vi "纳清浊度电极校准.vi"() -> ()   [LabVIEW 2016, in "斯坦道多参数.lvlib"]
uses:
  <vilib>/Utility/miscctls.llb/LVPointTypeDef.ctl
  <vilib>/Utility/miscctls.llb/LVPositionTypeDef.ctl
  <vilib>/Analysis/NI_AALBase.lvlib
panel:
  out "校准量程":u16(ring) items=["0-100", "0-500", "0-2000", "0-4000"]
  out "量程":u16(ring) items=["0-100", "0-500", "0-2000", "0-4000"]
  out "探头类别":string
  out "报警信息":string
  out "通讯状态":string
  out "温度校准参数":sgl
  out "第三点校准值":dbl
  out "标液3":sgl
  out "第二点校准值":dbl
  out "第一点校准值":dbl
  in  "校准停止":bool
  in  "校准启动":bool
  in  "校准模式":enum16{"两点校准", "单点校准", "三点校准"}(ring)=enum."单点校准"
  out "最小值":sgl format="%#.2f"
  out "最大值":sgl format="%#.2f"
  out "波形图表":u16(graph) caption="历史曲线"
  out "mean":dbl caption="均值" format="%#.2f"
  out "standard deviation":dbl caption="标准差" format="%#.2f"
  out "变异系数":dbl format="%#.6f"
  out "测量值":sgl
  out "提示":string
  out "标液2":sgl
  out "标液1":sgl
  out "原始光强数值":u16 caption="信号值"
  out "温度":dbl
  # "浊度电极设定"
  # "℃"
  # "NTU"
  # "NTU"
  # "NTU"
  # "℃"
  # "请选择校准模式:"
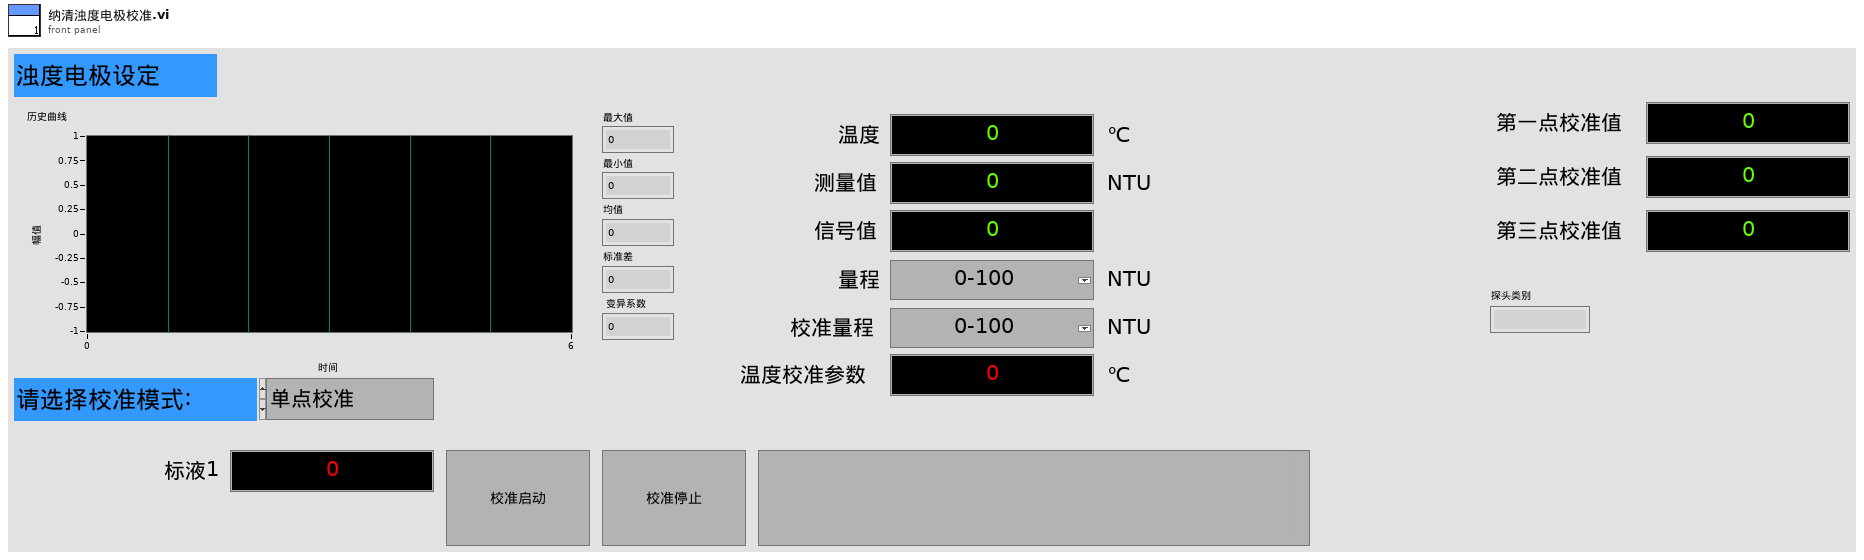
[diagram p1: front panel]
types:
  T1 = typedef "LVPointTypeDef.ctl" = cluster{"Horizontal":i16, "Vertical":i16}
  T2 = typedef "斯坦道多参数.lvlib/校准步骤.ctl" = enum16{"待机", "放置第一点标液", "第一点校准启动", "第一点校准写入", "第一点校准失败", "放置第二点标液", "第二点校准启动", "第二点校准写入", "第二点校准失败", "放置第三点标液", "第三点校准启动", "第三点校准写入", "第三点校准失败", "校准结果写入", "校准结束"}
  T3 = cluster{"报警码":u16, "浊度数值 NTU":sgl, "温度数据":sgl, "原始光强数值":u16, "量程":u16, "平均次数":u16, "清扫模式":u16, "清扫次数":u16, "清扫间隔分钟":u16, "0X000B_NC":string, "产品名称":string, "序列号":string, "硬件版本":string, "软件版本":string, "通讯地址":u16, "波特率":u16, "设备类型":u16, "0X0026_NC":string, "校准量程":u16, "第一点原始光强":u16, "第一点校准数据":sgl, "第二点原始光强":u16, "第二点校准数据":sgl, "第三点原始光强":u16, "第三点校准数据":sgl, "探头校准命令":u16, "温度校准参数":sgl, "温度校准命令":u16}
  T4 = typedef "LVPositionTypeDef.ctl" = cluster{"Left":i32, "Top":i32}
  T5 = cluster{"报警码":u16, "叶绿素a":sgl, "温度数据":sgl, "原始光强数值":u16, "0X0006_NC":u16, "平均次数":u16, "清扫模式":u16, "清扫次数":u16, "清扫间隔分钟":u16, "0X000B_NC":string, "产品名称":string, "序列号":string, "硬件版本":string, "软件版本":string, "通讯地址":u16, "波特率":u16, "设备类型":u16, "0X0026_NC":string, "0X0030_NC":u16, "第一点原始光强":u16, "第一点校准数据":sgl, "第二点原始光强":u16, "第二点校准数据":sgl, "第三点原始光强":u16, "第三点校准数据":sgl, "探头校准命令":u16, "温度校准参数":sgl, "温度校准命令":u16}
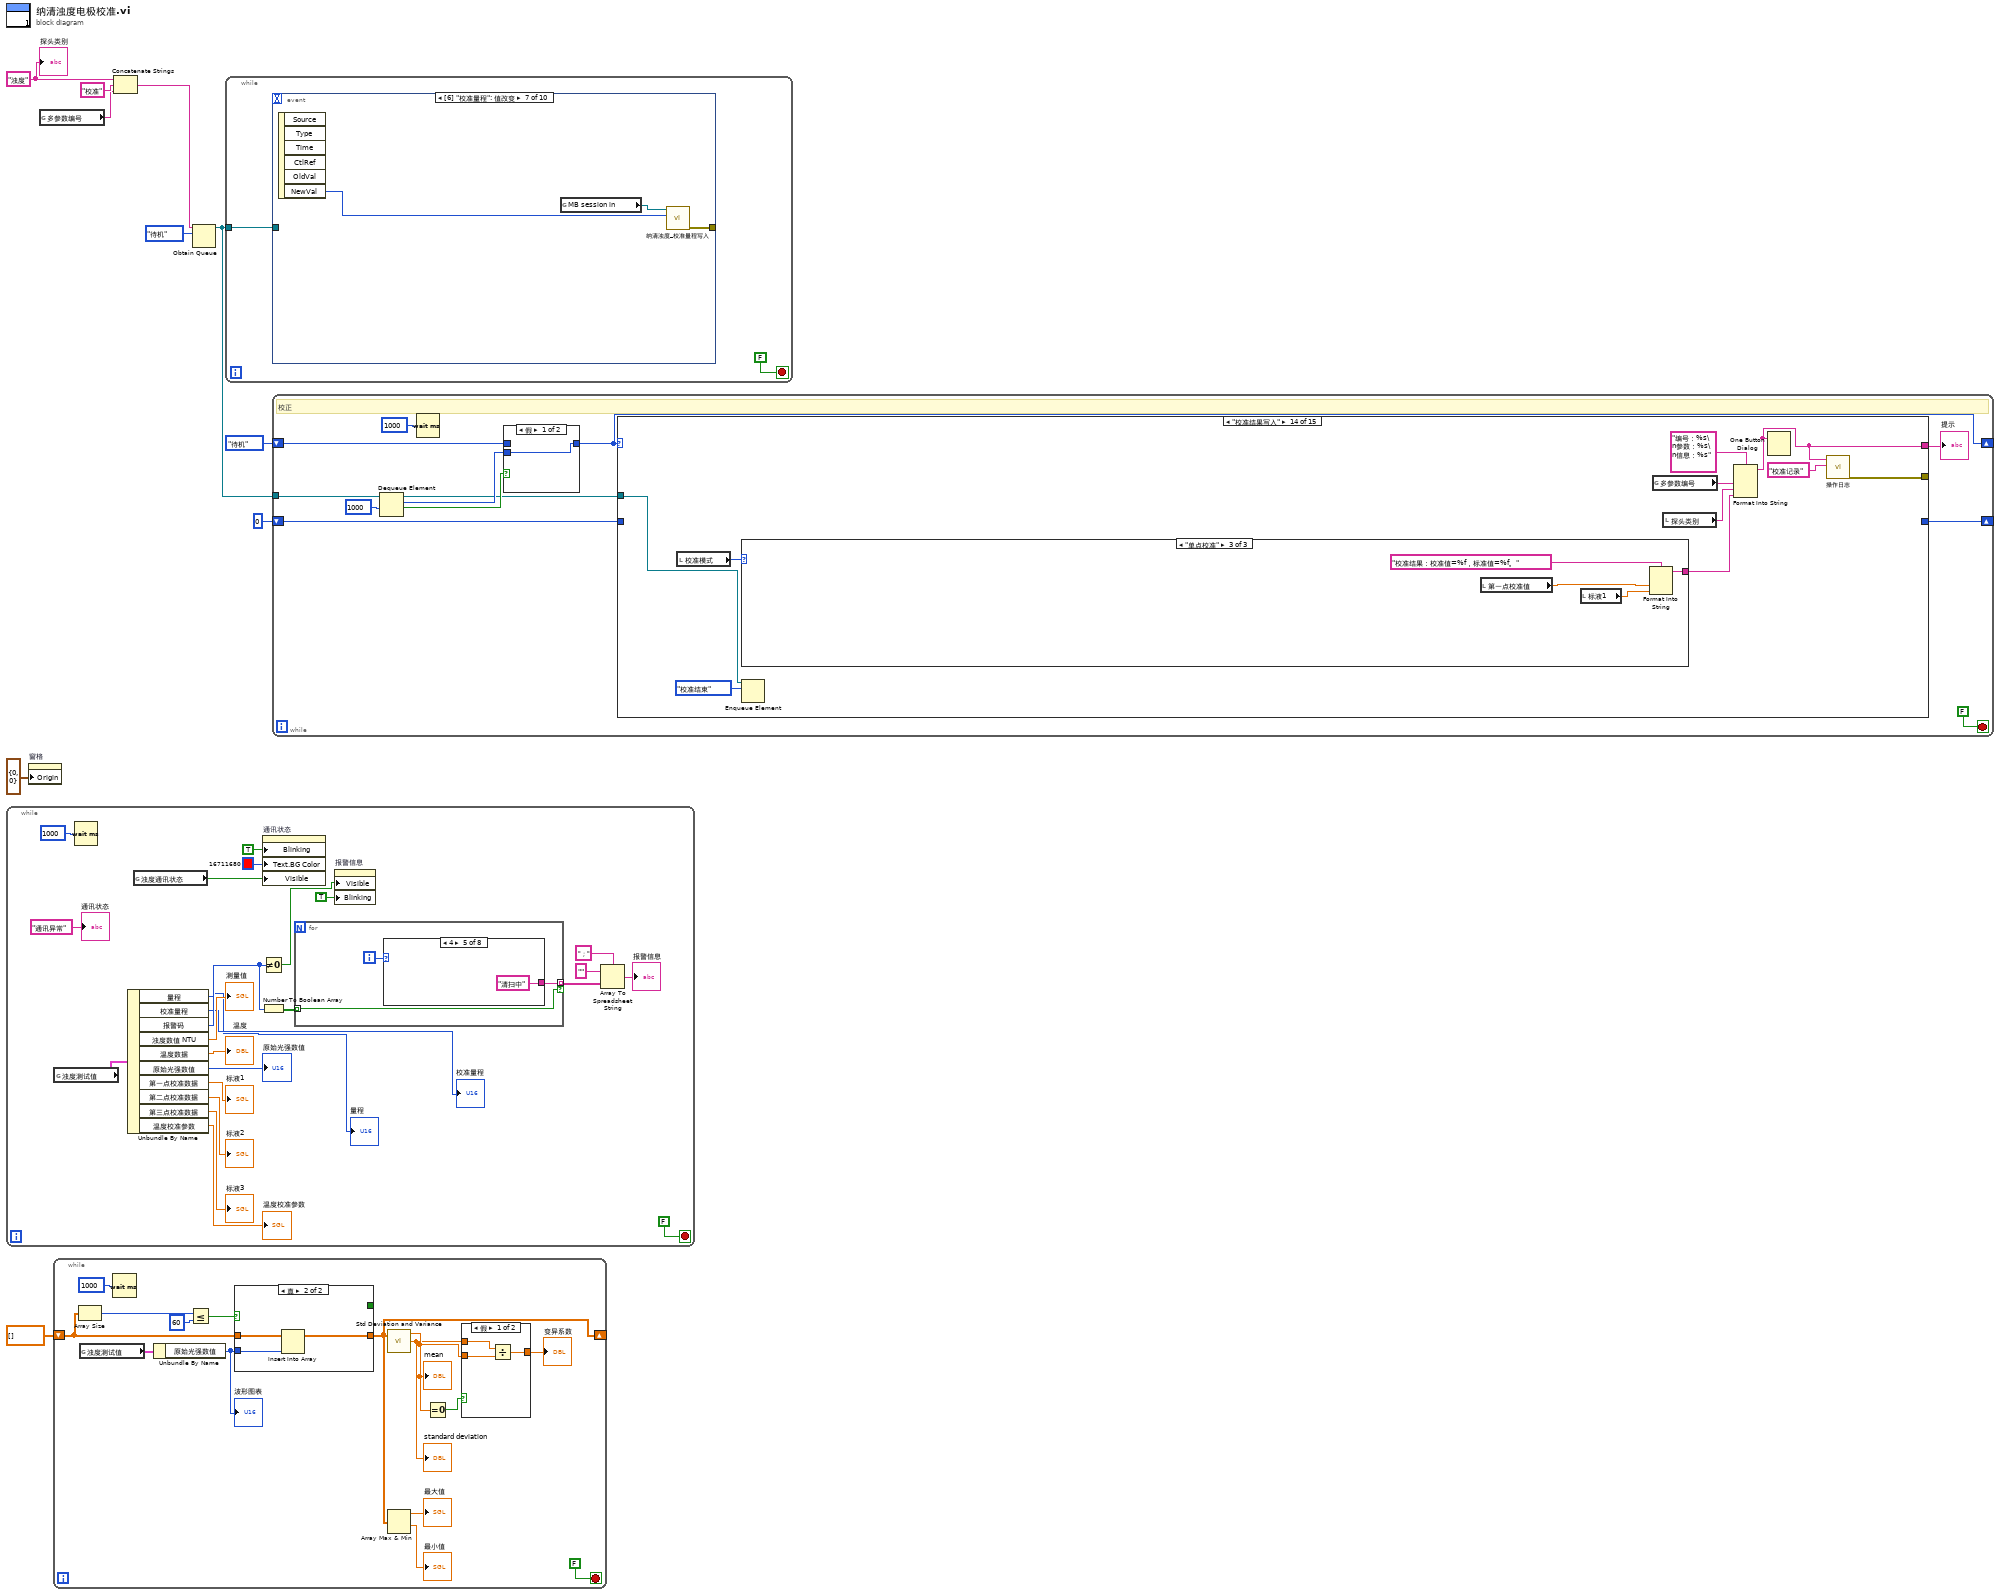
[diagram p0: block diagram]
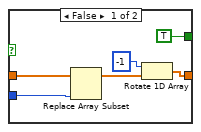
[diagram p3: hidden frame]
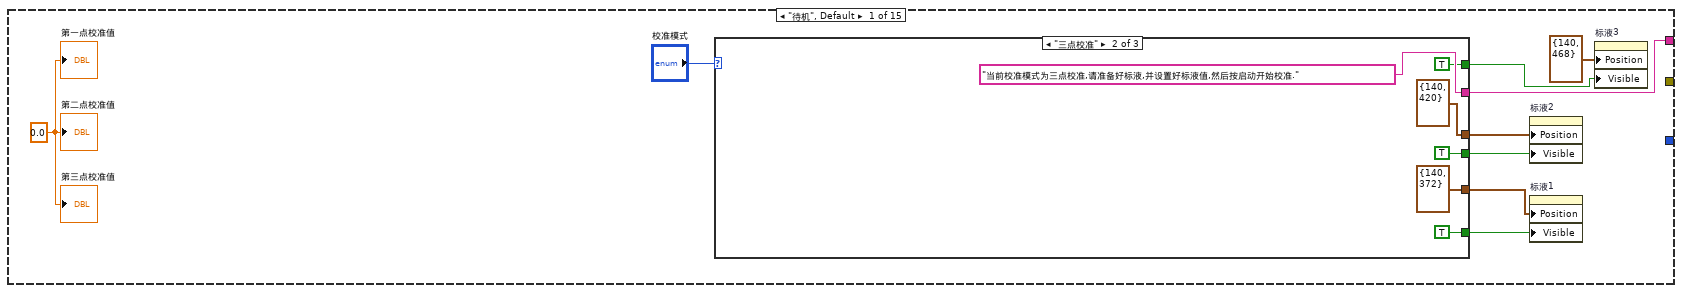
[diagram p5: hidden frame]
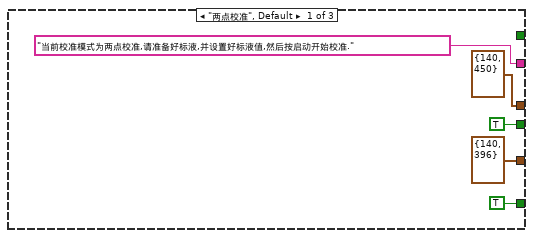
[diagram p6: hidden frame]
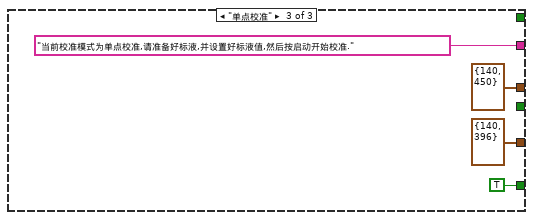
[diagram p7: hidden frame]
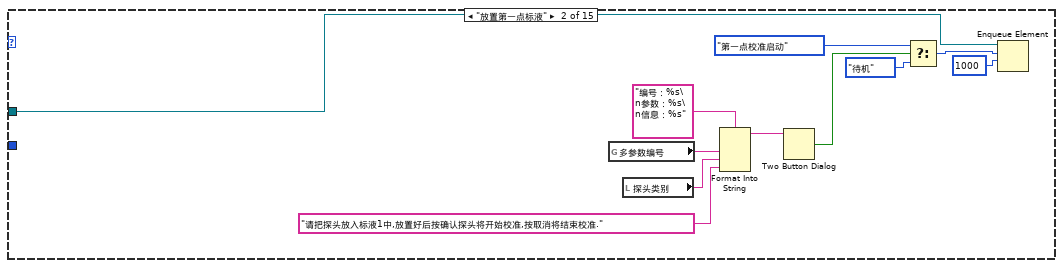
[diagram p8: hidden frame]
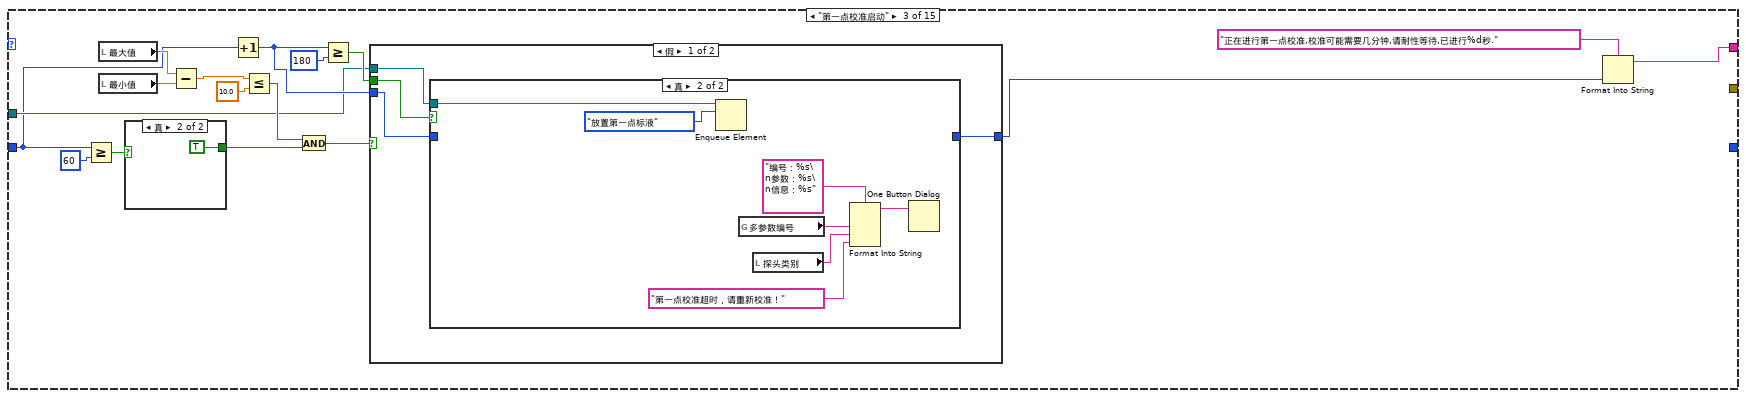
[diagram p9: hidden frame]
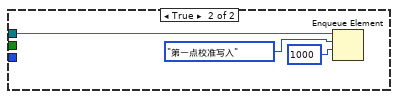
[diagram p11: hidden frame]
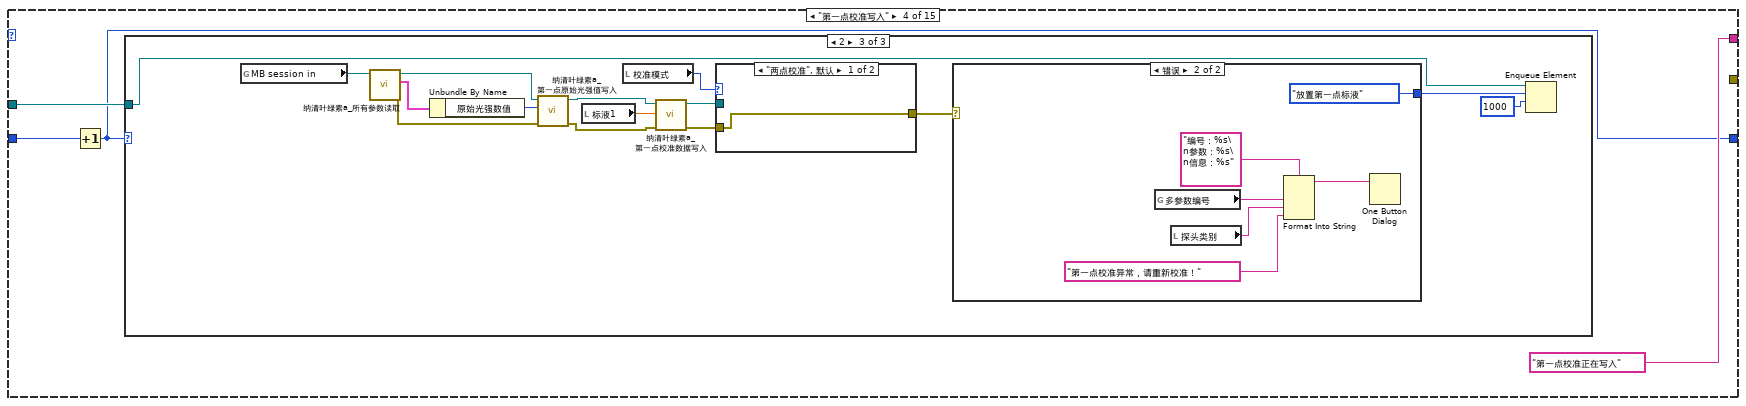
[diagram p13: hidden frame]
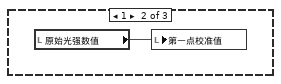
[diagram p15: hidden frame]
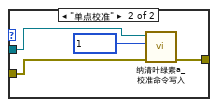
[diagram p16: hidden frame]
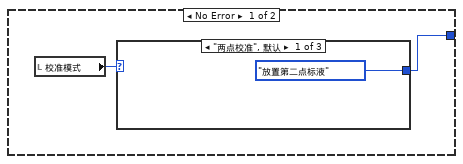
[diagram p17: hidden frame]
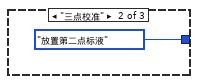
[diagram p18: hidden frame]
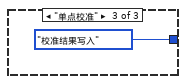
[diagram p19: hidden frame]
diagram:
  w1 = "浊度" ("名称（未命名）")
  n1 = while {
    stop <- FALSE stop-if-true
    n2 = global read "纳清过程全局变量.vi" "浊度测试值"() -> (w32:T3)
    n3 = Wait (ms)(milliseconds to wait=u32 1000 ("等待时间（毫秒）")) -> ()  [unwired: 1 out]
    n4 = Unbundle By Name(w32) -> ("量程"=→"量程":u16, "校准量程"=→"校准量程":u16, "报警码"=w13:u16, "浊度数值 NTU"=→"测量值":sgl, "温度数据"=→"温度":sgl, "原始光强数值"=→"原始光强数值":u16, "第一点校准数据"=→"标液1":sgl, "第二点校准数据"=→"标液2":sgl, "第三点校准数据"=→"标液3":sgl, "温度校准参数"=→"温度校准参数":sgl)
    n5 = global read "多参数全局变量.vi" "浊度通讯状态"() -> (w21:bool)
    n6 = Not Equal To 0?(x=w13) -> (x != 0?=w15:bool)
    n7 = Number To Boolean Array(number=w13) -> (Boolean array=w20:bool[])
    n8 = property on="通讯状态" class="Str"("Blinking"=TRUE ("闪烁"), "Text.BG Color"=u32 16711680, "Visible"=w21) -> ()  [unwired: 2 in, 2 out]
    n9 = for {
      tunnel: w20 -> [w35] mode=indexing
      tunnel: [w36] -> w19 mode=indexing if=w35
      i -> [w37]
      n10 = case shown="4" w37 {
        tunnel: [_ "浊度超量程" "温度超量程" "光强信号超范围" "清扫中" "温度传感器故障" "电极故障" "内部电压基准故障"] -> w36
        frame Default {
        }
        frame 0 {
        }
        frame 2 {
        }
        frame 3 {
        }
        frame 4 {
        }
        frame 8 {
        }
        frame 9 {
        }
        frame 10 {
        }
      }
    }
    n11 = property on="报警信息" class="Str"("Visible"=w15, "Blinking"=TRUE ("闪烁")) -> ()  [unwired: 2 in, 2 out]
    n12 = Array To Spreadsheet String(delimiter (Tab)="；" ("分隔符(Tab)"), array=w19, 3:"" ("格式字符串")) -> (spreadsheet string=→"报警信息":string)
    "通讯状态" <- "通讯异常" ("当前串口")
  }
  n13 = property on="窗格" class="Pane"("Origin"=T1 {"Horizontal"=0, "Vertical"=0} ("原点")) -> ()  [unwired: 2 in, 2 out]
  n14 = global read "多参数全局变量.vi" "多参数编号"() -> (w2:string)
  n15 = while {
    shift-right: [w49] -> _
    shift-left: sgl[] [] -> [w55]
    stop <- FALSE stop-if-true
    n16 = Array Size(array=w55) -> (size(s)=w57:i32)
    n17 = global read "纳清过程全局变量.vi" "浊度测试值"() -> (w45:T3)
    n18 = Wait (ms)(milliseconds to wait=u32 1000 ("等待时间（毫秒）")) -> ()  [unwired: 1 out]
    n19 = Unbundle By Name(w45) -> ("原始光强数值"=w46:u16)
    "波形图表" <- w46
    n20 = Less Or Equal?(x=w57, y=60) -> (x <= y?=w56:bool)
    n21 = case shown="真" w56 {
      tunnel: w55 -> [w68 w71]
      tunnel: w46 -> [w66 w70]
      tunnel: [w64 w69] -> w49
      tunnel: [TRUE _] -> _
      frame False {
        n22 = Replace Array Subset(array=w68, new element=w66) -> (w67:sgl[])  [unwired: 1 in]
        n23 = Rotate 1D Array(1:w67, 2:-1 ("n")) -> (0:w64:sgl[])
      }
      frame True {
        n24 = Insert Into Array(array=w71, new element=w70) -> (w69:sgl[])  [unwired: 1 in]
      }
    }
    n25 = call <vilib>:"Std Deviation and Variance.vi"("X"=w49) -> ("mean"=w53:dbl, "standard deviation"=w52:dbl)  [unwired: 1 in, 1 out]
    "mean" <- w53
    "standard deviation" <- w52
    n26 = Array Max & Min(array=w49) -> (max value=→"最大值":sgl, min value=→"最小值":sgl)  [unwired: 2 out]
    n27 = Equal To 0?(x=w53) -> (x = 0?=w54:bool)
    n28 = case shown="假" w54 {
      tunnel: w52 -> [w62 _]
      tunnel: [w61 _] -> w51
      tunnel: w53 -> [w60 _]
      frame False {
        n29 = Divide(x=w62, y=w60) -> (x/y=w61:dbl)
      }
      frame True {
      }
    }
    "变异系数" <- w51
  }
  n30 = Concatenate Strings(w1, "校准" ("名称（未命名）"), w2) -> (w3:string)
  n31 = Obtain Queue(name (unnamed)=w3, element data type=校准步骤."待机" ("枚举")) -> (queue out=w5:refnum<queue>)  [unwired: 3 in, 2 out]
  n32 = while {
    tunnel: w5 -> [w72]
    stop <- FALSE stop-if-true
    n33 = event shown="[6] \"校准量程\": 值改变" {
      selector: _ -> [_ _ _ _ _ _ _ _ _ _]
      dyn-events: _ -> [_ _ _ _ _ _ _ _ _ _]
      timeout: _ -> [_ _ _ _ _ _ _ _ _ _]
      tunnel: [_ _ w79 w83 w86 w89 w92 w93 _ _] -> _
      tunnel: w72 -> [_ _ _ _ _ _ _ _ w100 w102]
      event Timeout {
        n34 = event-data() -> ()  [unwired: 1 in, 3 out]
      }
      event "标液1", "标液2", "标液3", "温度校准参数": Mouse Down {
        n35 = event-data() -> ("CtlRef"=w74:refnum<vi>)  [unwired: 1 in, 7 out]
        n36 = property class="DigNum (严格)"(reference=w74) -> (reference out=w75:refnum<vi>, "Value"=w76:sgl)  [unwired: 1 in, 1 out]
        n37 = call "数字键盘.vi"("OldNumber"=w76) -> ("NewNumber"=w77:dbl)  [unwired: 1 in]
        n38 = property class="DigNum (严格)"(reference=w75, "Val(Sgnl)"=w77) -> ()  [unwired: 1 in, 2 out]
      }
      event "标液1": Value Change {
        n39 = event-data() -> ("NewVal"=w78:sgl)  [unwired: 1 in, 5 out]
        n40 = global read "多参数全局变量.vi" "MB session in"() -> (w80:refnum<class "MB_Master.lvclass">)
        n41 = call "纳清叶绿素a_第一点校准数据写入.vi"("数值"=w78, "MB session in"=w80) -> ("error out"=w79:errorcluster)  [unwired: 8 in, 1 out]
      }
      event "标液2": Value Change {
        n42 = event-data() -> ("NewVal"=w82:sgl)  [unwired: 1 in, 5 out]
        n43 = global read "多参数全局变量.vi" "MB session in"() -> (w81:refnum<class "MB_Master.lvclass">)
        n44 = call "纳清叶绿素a_第二点校准数据写入.vi"("数值"=w82, "MB session in"=w81) -> ("error out"=w83:errorcluster)  [unwired: 8 in, 1 out]
      }
      event "标液3": Value Change {
        n45 = event-data() -> ("NewVal"=w84:sgl)  [unwired: 1 in, 5 out]
        n46 = global read "多参数全局变量.vi" "MB session in"() -> (w85:refnum<class "MB_Master.lvclass">)
        n47 = call "纳清叶绿素a_第三点校准数据写入.vi"("数值"=w84, "MB session in"=w85) -> ("error out"=w86:errorcluster)  [unwired: 8 in, 1 out]
      }
      event "量程": Value Change {
        n48 = event-data() -> ("NewVal"=w87:u16)  [unwired: 1 in, 5 out]
        n49 = global read "多参数全局变量.vi" "MB session in"() -> (w88:refnum<class "MB_Master.lvclass">)
        n50 = call "纳清浊度_量程写入.vi"("数值"=w87, "MB session in"=w88) -> ("error out"=w89:errorcluster)  [unwired: 8 in, 1 out]
      }
      event "校准量程": Value Change {
        n51 = event-data() -> ("NewVal"=w90:u16)  [unwired: 1 in, 5 out]
        n52 = global read "多参数全局变量.vi" "MB session in"() -> (w91:refnum<class "MB_Master.lvclass">)
        n53 = call "纳清浊度_校准量程写入.vi"("数值"=w90, "MB session in"=w91) -> ("error out"=w92:errorcluster)  [unwired: 8 in, 1 out]
      }
      event "温度校准参数": Value Change {
        n54 = event-data() -> ("NewVal"=w98:sgl)  [unwired: 1 in, 5 out]
        n55 = global read "多参数全局变量.vi" "MB session in"() -> (w97:refnum<class "MB_Master.lvclass">)
        n56 = call "纳清叶绿素a_温度校准参数写入.vi"("数值"=w98, "MB session in"=w97) -> ("error out"=w99:errorcluster, "MB session out"=w96:refnum<class "MB_Master.lvclass">)  [unwired: 8 in]
        n57 = call "纳清叶绿素a_温度校准命令写入.vi"("error in (no error)"=w99, "数值"=u16 1 ("starting address"), "MB session in"=w96) -> ("error out"=w94:errorcluster)  [unwired: 7 in, 1 out]
        n58 = call <vilib>:"Simple Error Handler.vi"("error in (no error)"=w94) -> ("error out"=w93:errorcluster)  [unwired: 4 in, 4 out]
      }
      event "校准启动": Value Change {
        n59 = event-data() -> ()  [unwired: 1 in, 6 out]
        n60 = Enqueue Element(queue=w100, element=校准步骤."放置第一点标液" ("元素")) -> ()  [unwired: 2 in, 3 out]
      }
      event "校准停止": Value Change {
        n61 = event-data() -> ()  [unwired: 1 in, 6 out]
        n62 = Flush Queue(queue=w102) -> (queue out=w103:refnum<queue>)  [unwired: 1 in, 2 out]
        n63 = Enqueue Element(queue=w103, element=校准步骤."待机" ("元素"), timeout in ms (-1)=1000 ("超时毫秒(-1)")) -> ()  [unwired: 1 in, 3 out]
      }
    }
  }
  n64 = while "While循环" {
    shift-right: [w107] -> _
    shift-left: 校准步骤."待机" ("枚举") -> [w109]
    shift-right: [w106] -> _
    shift-left: 0 -> [w115]
    tunnel: w5 -> [w110]
    stop <- FALSE stop-if-true
    # "校正"
    n65 = Dequeue Element(queue=w110, timeout in ms (-1)=1000 ("超时毫秒(-1)")) -> (queue out=w108:refnum<queue>, element=w111:T2, timed out?=w112:bool)  [unwired: 1 in, 1 out]
    n66 = Wait (ms)(milliseconds to wait=u32 1000 ("等待时间（毫秒）")) -> ()  [unwired: 1 out]
    n67 = case shown="假" w112 {
      tunnel: w111 -> [w118 _]
      tunnel: [w118 w119] -> w107
      tunnel: w109 -> [_ w119]
      frame False {
      }
      frame True {
      }
    }
    n68 = case shown="\"校准结果写入\"" w107 {
      tunnel: [w127 _ w155 "第一点校准正在写入" ("提示") _ _ w237 "第二点校准正在写入" ("提示") "第二点校准失败" ("提示") _ "第三点校准正在写入" ("提示") w349 "第三点校准失败" ("提示") w383 w409] -> w114
      tunnel: w115 -> [_ _ w157 w190 _ _ w238 w270 _ _ w318 w350 _ _ _]
      tunnel: [_ _ _ w188 _ _ w236 w268 _ _ w316 w348 _ _ _] -> w106
      tunnel: w108 -> [_ w150 w158 w189 _ w229 w239 w269 _ w310 w317 w351 _ w389 _]
      tunnel: [_ _ _ _ _ _ _ _ _ _ _ _ _ w387 _] -> _
      frame "待机", Default {
        w120 = 0.0 ("第一点校准值")
        n69 = case shown="\"三点校准\"" "校准模式" {
          tunnel: ["当前校准模式为两点校准,请准备好标液,并设置好标液值,然后按启动开始校准." ("提示") "当前校准模式为三点校准,请准备好标液,并设置好标液值,然后按启动开始校准." ("提示") "当前校准模式为单点校准,请准备好标液,并设置好标液值,然后按启动开始校准." ("提示")] -> w127
          tunnel: [TRUE ("可见") TRUE ("可见") _] -> w123
          tunnel: [T4 {"Left"=140, "Top"=396} ("位置") T4 {"Left"=140, "Top"=372} ("位置") T4 {"Left"=140, "Top"=396} ("位置")] -> w126
          tunnel: [T4 {"Left"=140, "Top"=450} ("位置 2") T4 {"Left"=140, "Top"=420} ("位置 2") T4 {"Left"=140, "Top"=450} ("位置 2")] -> w125
          tunnel: [_ TRUE ("可见") _] -> w122
          tunnel: [TRUE ("可见") TRUE ("可见") TRUE ("可见")] -> w121
          frame "两点校准", Default {
          }
          frame "三点校准" {
          }
          frame "单点校准" {
          }
        }
        n70 = property on="标液2" class="DigNum (严格)"("Position"=w125, "Visible"=w123) -> ()  [unwired: 2 in, 2 out]
        n71 = property on="标液1" class="DigNum (严格)"("Position"=w126, "Visible"=w121) -> ()  [unwired: 2 in, 2 out]
        n72 = property on="标液3" class="DigNum (严格)"("Position"=T4 {"Left"=140, "Top"=468} ("位置 3"), "Visible"=w122) -> ()  [unwired: 2 in, 2 out]
        "第一点校准值" <- w120
        "第二点校准值" <- w120
        "第三点校准值" <- w120
      }
      frame "放置第一点标液" {
        n73 = global read "多参数全局变量.vi" "多参数编号"() -> (w148:string)
        n74 = local read "探头类别"() -> (w144:string)
        n75 = Format Into String(format string="编号：%s\n参数：%s\n信息：%s" ("格式字符串"), w148, w144, "请把探头放入标液1中,放置好后按确认探头将开始校准,按取消将结束校准." ("消息")) -> (resulting string=w147:string)  [unwired: 2 in, 1 out]
        n76 = Two Button Dialog(message=w147) -> (T button?=w145:bool)  [unwired: 2 in]
        n77 = Select(t=校准步骤."第一点校准启动" ("元素"), s=w145, f=校准步骤."待机" ("元素")) -> (s? t:f=w151:T2)
        n78 = Enqueue Element(queue=w150, element=w151, timeout in ms (-1)=1000 ("超时毫秒(-1)")) -> ()  [unwired: 1 in, 3 out]
      }
      frame "第一点校准启动" {
        n79 = Greater Or Equal?(x=w157, y=60) -> (x >= y?=w164:bool)
        n80 = local read "最大值"() -> (w167:sgl)
        n81 = local read "最小值"() -> (w166:sgl)
        n82 = case shown="真" w164 {
          tunnel: [_ TRUE] -> w165
          frame False {
          }
          frame True {
          }
        }
        n83 = Subtract(x=w167, y=w166) -> (x-y=w168:sgl)
        n84 = Increment(x=w157) -> (x+1=w171:i32)
        n85 = Less Or Equal?(x=w168, y=10.0) -> (x <= y?=w161:bool)
        n86 = And(x=w161, y=w165) -> (x .and. y?=w169:bool)
        n87 = Greater Or Equal?(x=w171, y=180) -> (x >= y?=w170:bool)
        n88 = case shown="假" w169 {
          tunnel: w158 -> [w174 w186]
          tunnel: w170 -> [w175 _]
          tunnel: w171 -> [w173 _]
          tunnel: [w172 _] -> w156
          frame False {
            n89 = case shown="真" w175 {
              tunnel: w174 -> [_ w183]
              tunnel: w173 -> [w176 _]
              tunnel: [w176 _] -> w172
              frame False {
              }
              frame True {
                n90 = Enqueue Element(queue=w183, element=校准步骤."放置第一点标液" ("元素")) -> ()  [unwired: 2 in, 3 out]
                n91 = global read "多参数全局变量.vi" "多参数编号"() -> (w180:string)
                n92 = local read "探头类别"() -> (w177:string)
                n93 = Format Into String(format string="编号：%s\n参数：%s\n信息：%s" ("格式字符串"), w180, w177, "第一点校准超时，请重新校准！" ("error source (\" \")")) -> (resulting string=w178:string)  [unwired: 2 in, 1 out]
                n94 = One Button Dialog(message=w178) -> ()  [unwired: 1 in, 1 out]
              }
            }
          }
          frame True {
            n95 = Enqueue Element(queue=w186, element=校准步骤."第一点校准写入" ("元素"), timeout in ms (-1)=1000 ("超时毫秒(-1)")) -> ()  [unwired: 1 in, 3 out]
          }
        }
        n96 = Format Into String(format string="正在进行第一点校准,校准可能需要几分钟,请耐性等待,已进行%d秒." ("格式字符串"), w156) -> (resulting string=w155:string)  [unwired: 2 in, 1 out]
      }
      frame "第一点校准写入" {
        n97 = Increment(x=w190) -> (x+1=w188:i32)
        n98 = case shown="2" w188 {
          tunnel: w189 -> [_ _ w207]
          frame 0, Default {
          }
          frame 1 {
            n99 = local read "原始光强数值"() -> (w192:u16)
            n100 = local write "第一点校准值"(w192) -> ()
          }
          frame 2 {
            n101 = global read "多参数全局变量.vi" "MB session in"() -> (w203:refnum<class "MB_Master.lvclass">)
            n102 = call "纳清叶绿素a_所有参数读取.vi"("MB session in"=w203) -> ("error out"=w205:errorcluster, "输出值"=w202:T5, "MB session out"=w204:refnum<class "MB_Master.lvclass">)  [unwired: 8 in]
            n103 = Unbundle By Name(w202) -> ("原始光强数值"=w201:u16)
            n104 = call "纳清叶绿素a_第一点原始光强值写入.vi"("error in (no error)"=w205, "数值"=w201, "MB session in"=w204) -> ("error out"=w200:errorcluster, "MB session out"=w199:refnum<class "MB_Master.lvclass">)  [unwired: 7 in]
            n105 = local read "标液1"() -> (w196:sgl)
            n106 = local read "校准模式"() -> (w193:enum16{"两点校准", "单点校准", "三点校准"})
            n107 = call "纳清叶绿素a_第一点校准数据写入.vi"("error in (no error)"=w200, "数值"=w196, "MB session in"=w199) -> ("error out"=w198:errorcluster, "MB session out"=w197:refnum<class "MB_Master.lvclass">)  [unwired: 7 in]
            n108 = case shown="\"两点校准\", 默认" w193 {
              tunnel: w198 -> [w208 w212]
              tunnel: w197 -> [_ w211]
              tunnel: [w208 w209] -> w195
              frame "两点校准", Default {
              }
              frame "单点校准" {
                n109 = call "纳清叶绿素a_校准命令写入.vi"("error in (no error)"=w212, "数值"=u16 1 ("starting address"), "MB session in"=w211) -> ("error out"=w209:errorcluster)  [unwired: 7 in, 1 out]
              }
            }
            n110 = case shown="错误" w195 {
              tunnel: [w213 校准步骤."放置第一点标液" ("元素")] -> w194
              frame No Error {
                n111 = local read "校准模式"() -> (w214:enum16{"两点校准", "单点校准", "三点校准"})
                n112 = case shown="\"两点校准\", 默认" w214 {
                  tunnel: [校准步骤."放置第二点标液" ("元素") 校准步骤."放置第二点标液" ("元素") 校准步骤."校准结果写入" ("元素")] -> w213
                  frame "两点校准", Default {
                  }
                  frame "三点校准" {
                  }
                  frame "单点校准" {
                  }
                }
              }
              frame Error {
                n113 = global read "多参数全局变量.vi" "多参数编号"() -> (w222:string)
                n114 = local read "探头类别"() -> (w218:string)
                n115 = Format Into String(format string="编号：%s\n参数：%s\n信息：%s" ("格式字符串"), w222, w218, "第一点校准异常，请重新校准！" ("error source (\" \")")) -> (resulting string=w220:string)  [unwired: 2 in, 1 out]
                n116 = One Button Dialog(message=w220) -> ()  [unwired: 1 in, 1 out]
              }
            }
            n117 = Enqueue Element(queue=w207, element=w194, timeout in ms (-1)=1000 ("超时毫秒(-1)")) -> ()  [unwired: 1 in, 3 out]
          }
        }
      }
      frame "第一点校准失败" {
      }
      frame "放置第二点标液" {
        n118 = global read "多参数全局变量.vi" "多参数编号"() -> (w227:string)
        n119 = local read "探头类别"() -> (w224:string)
        n120 = Format Into String(format string="编号：%s\n参数：%s\n信息：%s" ("格式字符串"), w227, w224, "请把探头放入标液2中,放置好后按确认将继续校准,按取消将结束校准." ("消息")) -> (resulting string=w226:string)  [unwired: 2 in, 1 out]
        n121 = Two Button Dialog(message=w226) -> (T button?=w233:bool)  [unwired: 2 in]
        n122 = Select(t=校准步骤."第二点校准启动" ("元素"), s=w233, f=校准步骤."待机" ("元素")) -> (s? t:f=w230:T2)
        n123 = Enqueue Element(queue=w229, element=w230, timeout in ms (-1)=1000 ("超时毫秒(-1)")) -> ()  [unwired: 1 in, 3 out]
      }
      frame "第二点校准启动" {
        n124 = Greater Or Equal?(x=w238, y=60) -> (x >= y?=w244:bool)
        n125 = local read "最大值"() -> (w247:sgl)
        n126 = local read "最小值"() -> (w246:sgl)
        n127 = case shown="真" w244 {
          tunnel: [_ TRUE] -> w245
          frame False {
          }
          frame True {
          }
        }
        n128 = Subtract(x=w247, y=w246) -> (x-y=w248:sgl)
        n129 = Increment(x=w238) -> (x+1=w251:i32)
        n130 = Less Or Equal?(x=w248, y=10.0) -> (x <= y?=w241:bool)
        n131 = And(x=w241, y=w245) -> (x .and. y?=w249:bool)
        n132 = Greater Or Equal?(x=w251, y=180) -> (x >= y?=w250:bool)
        n133 = case shown="假" w249 {
          tunnel: w239 -> [w254 w266]
          tunnel: w250 -> [w255 _]
          tunnel: w251 -> [w253 _]
          tunnel: [w252 _] -> w236
          frame False {
            n134 = case shown="真" w255 {
              tunnel: w254 -> [_ w263]
              tunnel: w253 -> [w256 _]
              tunnel: [w256 _] -> w252
              frame False {
              }
              frame True {
                n135 = Enqueue Element(queue=w263, element=校准步骤."放置第二点标液" ("元素")) -> ()  [unwired: 2 in, 3 out]
                n136 = global read "多参数全局变量.vi" "多参数编号"() -> (w260:string)
                n137 = local read "探头类别"() -> (w257:string)
                n138 = Format Into String(format string="编号：%s\n参数：%s\n信息：%s" ("格式字符串"), w260, w257, "第二点校准超时，请重新校准！" ("消息")) -> (resulting string=w259:string)  [unwired: 2 in, 1 out]
                n139 = One Button Dialog(message=w259) -> ()  [unwired: 1 in, 1 out]
              }
            }
          }
          frame True {
            n140 = Enqueue Element(queue=w266, element=校准步骤."第二点校准写入" ("元素"), timeout in ms (-1)=1000 ("超时毫秒(-1)")) -> ()  [unwired: 1 in, 3 out]
          }
        }
        n141 = Format Into String(format string="正在进行第二点校准,校准可能需要几分钟,请耐性等待,已进行%d秒." ("格式字符串"), w236) -> (resulting string=w237:string)  [unwired: 2 in, 1 out]
      }
      frame "第二点校准写入" {
        n142 = Increment(x=w270) -> (x+1=w268:i32)
        n143 = case shown="2" w268 {
          tunnel: w269 -> [_ _ w287]
          frame 0, Default {
          }
          frame 1 {
            n144 = local read "原始光强数值"() -> (w272:u16)
            n145 = local write "第二点校准值"(w272) -> ()
          }
          frame 2 {
            n146 = global read "多参数全局变量.vi" "MB session in"() -> (w283:refnum<class "MB_Master.lvclass">)
            n147 = call "纳清叶绿素a_所有参数读取.vi"("MB session in"=w283) -> ("error out"=w285:errorcluster, "输出值"=w282:T5, "MB session out"=w284:refnum<class "MB_Master.lvclass">)  [unwired: 8 in]
            n148 = Unbundle By Name(w282) -> ("原始光强数值"=w281:u16)
            n149 = call "纳清叶绿素a_第二点原始光强值写入.vi"("error in (no error)"=w285, "数值"=w281, "MB session in"=w284) -> ("error out"=w280:errorcluster, "MB session out"=w279:refnum<class "MB_Master.lvclass">)  [unwired: 7 in]
            n150 = local read "标液2"() -> (w276:sgl)
            n151 = local read "校准模式"() -> (w273:enum16{"两点校准", "单点校准", "三点校准"})
            n152 = call "纳清叶绿素a_第二点校准数据写入.vi"("error in (no error)"=w280, "数值"=w276, "MB session in"=w279) -> ("error out"=w278:errorcluster, "MB session out"=w277:refnum<class "MB_Master.lvclass">)  [unwired: 7 in]
            n153 = case shown="\"单点校准\", 默认" w273 {
              tunnel: w278 -> [w291 w292]
              tunnel: w277 -> [w290 _]
              tunnel: [w288 w292] -> w275
              frame "两点校准" {
                n154 = call "纳清叶绿素a_校准命令写入.vi"("error in (no error)"=w291, "数值"=u16 2 ("starting address"), "MB session in"=w290) -> ("error out"=w288:errorcluster)  [unwired: 7 in, 1 out]
              }
              frame "单点校准", Default {
              }
            }
            n155 = case shown="错误" w275 {
              tunnel: [w293 校准步骤."放置第二点标液" ("元素")] -> w274
              frame No Error {
                n156 = local read "校准模式"() -> (w294:enum16{"两点校准", "单点校准", "三点校准"})
                n157 = case shown="\"两点校准\", 默认" w294 {
                  tunnel: [校准步骤."校准结果写入" ("元素") 校准步骤."放置第三点标液" ("元素") 校准步骤."校准结果写入" ("元素")] -> w293
                  frame "两点校准", Default {
                  }
                  frame "三点校准" {
                  }
                  frame "单点校准" {
                  }
                }
              }
              frame Error {
                n158 = global read "多参数全局变量.vi" "多参数编号"() -> (w302:string)
                n159 = local read "探头类别"() -> (w298:string)
                n160 = Format Into String(format string="编号：%s\n参数：%s\n信息：%s" ("格式字符串"), w302, w298, "第二点校准异常，请重新校准！" ("error source (\" \")")) -> (resulting string=w300:string)  [unwired: 2 in, 1 out]
                n161 = One Button Dialog(message=w300) -> ()  [unwired: 1 in, 1 out]
              }
            }
            n162 = Enqueue Element(queue=w287, element=w274, timeout in ms (-1)=1000 ("超时毫秒(-1)")) -> ()  [unwired: 1 in, 3 out]
          }
        }
      }
      frame "第二点校准失败" {
      }
      frame "放置第三点标液" {
        n163 = global read "多参数全局变量.vi" "多参数编号"() -> (w308:string)
        n164 = local read "探头类别"() -> (w305:string)
        n165 = Format Into String(format string="编号：%s\n参数：%s\n信息：%s" ("格式字符串"), w308, w305, "请把探头放入标液3中,放置好后按确认将继续校准,按取消将结束校准." ("消息")) -> (resulting string=w307:string)  [unwired: 2 in, 1 out]
        n166 = Two Button Dialog(message=w307) -> (T button?=w314:bool)  [unwired: 2 in]
        n167 = Select(t=校准步骤."第三点校准启动" ("元素"), s=w314, f=校准步骤."待机" ("元素")) -> (s? t:f=w311:T2)
        n168 = Enqueue Element(queue=w310, element=w311, timeout in ms (-1)=1000 ("超时毫秒(-1)")) -> ()  [unwired: 1 in, 3 out]
      }
      frame "第三点校准写入" {
        n169 = Increment(x=w318) -> (x+1=w316:i32)
        n170 = case shown="2" w316 {
          tunnel: w317 -> [_ _ w322]
          frame 0, Default {
          }
          frame 1 {
            n171 = local read "原始光强数值"() -> (w320:u16)
            n172 = local write "第二点校准值"(w320) -> ()
          }
          frame 2 {
            n173 = global read "多参数全局变量.vi" "MB session in"() -> (w333:refnum<class "MB_Master.lvclass">)
            n174 = call "纳清叶绿素a_所有参数读取.vi"("MB session in"=w333) -> ("error out"=w335:errorcluster, "输出值"=w332:T5, "MB session out"=w334:refnum<class "MB_Master.lvclass">)  [unwired: 8 in]
            n175 = Unbundle By Name(w332) -> ("原始光强数值"=w331:u16)
            n176 = call "纳清叶绿素a_第三点原始光强值写入.vi"("error in (no error)"=w335, "数值"=w331, "MB session in"=w334) -> ("error out"=w330:errorcluster, "MB session out"=w329:refnum<class "MB_Master.lvclass">)  [unwired: 7 in]
            n177 = local read "标液3"() -> (w325:sgl)
            n178 = call "纳清叶绿素a_第三点校准数据写入.vi"("error in (no error)"=w330, "数值"=w325, "MB session in"=w329) -> ("error out"=w328:errorcluster, "MB session out"=w327:refnum<class "MB_Master.lvclass">)  [unwired: 7 in]
            n179 = call "纳清叶绿素a_校准命令写入.vi"("error in (no error)"=w328, "数值"=u16 3 ("starting address"), "MB session in"=w327) -> ("error out"=w324:errorcluster)  [unwired: 7 in, 1 out]
            n180 = case shown="错误" w324 {
              tunnel: [w336 校准步骤."放置第三点标液" ("元素")] -> w321
              frame No Error {
                n181 = local read "校准模式"() -> (w337:enum16{"两点校准", "单点校准", "三点校准"})
                n182 = case shown="\"单点校准\"" w337 {
                  tunnel: [校准步骤."放置第二点标液" ("元素") 校准步骤."校准结果写入" ("元素") 校准步骤."校准结果写入" ("元素")] -> w336
                  frame "两点校准", Default {
                  }
                  frame "三点校准" {
                  }
                  frame "单点校准" {
                  }
                }
              }
              frame Error {
                n183 = global read "多参数全局变量.vi" "多参数编号"() -> (w345:string)
                n184 = local read "探头类别"() -> (w341:string)
                n185 = Format Into String(format string="编号：%s\n参数：%s\n信息：%s" ("格式字符串"), w345, w341, "第三点校准异常，请重新校准！" ("error source (\" \")")) -> (resulting string=w343:string)  [unwired: 2 in, 1 out]
                n186 = One Button Dialog(message=w343) -> ()  [unwired: 1 in, 1 out]
              }
            }
            n187 = Enqueue Element(queue=w322, element=w321, timeout in ms (-1)=1000 ("超时毫秒(-1)")) -> ()  [unwired: 1 in, 3 out]
          }
        }
      }
      frame "第三点校准启动" {
        n188 = Greater Or Equal?(x=w350, y=60) -> (x >= y?=w356:bool)
        n189 = local read "最大值"() -> (w359:sgl)
        n190 = local read "最小值"() -> (w358:sgl)
        n191 = case shown="真" w356 {
          tunnel: [_ TRUE] -> w357
          frame False {
          }
          frame True {
          }
        }
        n192 = Subtract(x=w359, y=w358) -> (x-y=w360:sgl)
        n193 = Increment(x=w350) -> (x+1=w363:i32)
        n194 = Less Or Equal?(x=w360, y=10.0) -> (x <= y?=w353:bool)
        n195 = And(x=w353, y=w357) -> (x .and. y?=w361:bool)
        n196 = Greater Or Equal?(x=w363, y=180) -> (x >= y?=w362:bool)
        n197 = case shown="假" w361 {
          tunnel: w351 -> [w366 w378]
          tunnel: w362 -> [w367 _]
          tunnel: w363 -> [w365 _]
          tunnel: [w364 _] -> w348
          frame False {
            n198 = case shown="真" w367 {
              tunnel: w366 -> [_ w375]
              tunnel: w365 -> [w368 _]
              tunnel: [w368 _] -> w364
              frame False {
              }
              frame True {
                n199 = Enqueue Element(queue=w375, element=校准步骤."放置第三点标液" ("元素")) -> ()  [unwired: 2 in, 3 out]
                n200 = global read "多参数全局变量.vi" "多参数编号"() -> (w372:string)
                n201 = local read "探头类别"() -> (w369:string)
                n202 = Format Into String(format string="编号：%s\n参数：%s\n信息：%s" ("格式字符串"), w372, w369, "第三点校准异常，请重新校准！" ("error source (\" \")")) -> (resulting string=w370:string)  [unwired: 2 in, 1 out]
                n203 = One Button Dialog(message=w370) -> ()  [unwired: 1 in, 1 out]
              }
            }
          }
          frame True {
            n204 = Enqueue Element(queue=w378, element=校准步骤."第三点校准写入" ("元素"), timeout in ms (-1)=1000 ("超时毫秒(-1)")) -> ()  [unwired: 1 in, 3 out]
          }
        }
        n205 = Format Into String(format string="正在进行第三点校准,校准可能需要几分钟,请耐性等待,已进行%d秒." ("格式字符串"), w348) -> (resulting string=w349:string)  [unwired: 2 in, 1 out]
      }
      frame "第三点校准失败" {
      }
      frame "校准结果写入" {
        n206 = local read "校准模式"() -> (w388:enum16{"两点校准", "单点校准", "三点校准"})
        n207 = case shown="\"单点校准\"" w388 {
          tunnel: [w393 w401 w408] -> w384
          frame "两点校准", Default {
            n208 = local read "第一点校准值"() -> (w396:dbl)
            n209 = local read "第二点校准值"() -> (w392:dbl)
            n210 = local read "标液1"() -> (w394:sgl)
            n211 = local read "标液2"() -> (w391:sgl)
            n212 = Format Into String(format string="校准结果：第一点校准值=%f，第一点标准值=%f,第二点校准值=%f，第二点标准值=%f." ("提示"), w396, w394, w392, w391) -> (resulting string=w393:string)  [unwired: 2 in, 1 out]
          }
          frame "三点校准" {
            n213 = local read "第一点校准值"() -> (w404:dbl)
            n214 = local read "第二点校准值"() -> (w400:dbl)
            n215 = local read "第三点校准值"() -> (w398:dbl)
            n216 = local read "标液1"() -> (w402:sgl)
            n217 = local read "标液2"() -> (w399:sgl)
            n218 = local read "标液3"() -> (w397:sgl)
            n219 = Format Into String(format string="校准结果：第一点校准值=%f，第一点标准值=%f,第二点校准值=%f，第二点标准值=%f,第三点校准值=%f，第三点标准值=%f." ("提示"), w404, w402, w400, w399, w398, w397) -> (resulting string=w401:string)  [unwired: 2 in, 1 out]
          }
          frame "单点校准" {
            n220 = local read "第一点校准值"() -> (w407:dbl)
            n221 = local read "标液1"() -> (w405:sgl)
            n222 = Format Into String(format string="校准结果：校准值=%f，标准值=%f。" ("提示"), w407, w405) -> (resulting string=w408:string)  [unwired: 2 in, 1 out]
          }
        }
        n223 = Enqueue Element(queue=w389, element=校准步骤."校准结束" ("元素")) -> ()  [unwired: 2 in, 3 out]
        n224 = global read "多参数全局变量.vi" "多参数编号"() -> (w385:string)
        n225 = local read "探头类别"() -> (w381:string)
        n226 = Format Into String(format string="编号：%s\n参数：%s\n信息：%s" ("格式字符串"), w385, w381, w384) -> (resulting string=w383:string)  [unwired: 2 in, 1 out]
        n227 = One Button Dialog(message=w383) -> ()  [unwired: 1 in, 1 out]
        n228 = call "操作日志.vi"("table"="校准记录", "日志信息"=w383) -> ("error out"=w387:errorcluster)  [unwired: 9 in]
      }
      frame "校准结束" {
        n229 = local read "提示"() -> (w409:string)
      }
    }
    "提示" <- w114
  }
  "探头类别" <- w1
